vi "Close Notifiers.vi"(8 "error in":errorcluster, 11 "Notifiers":T1) -> (0 "error out":errorcluster)   [LabVIEW 2015, in "Notifiers.lvlib"]
doc: "Releases notifiers"
uses:
  Notifiers.lvlib
  Notifiers.ctl
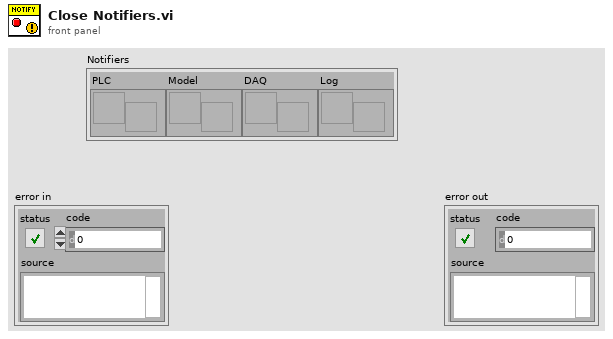
[diagram p1: front panel]
types:
  T1 = typedef "Notifiers.lvlib/Notifiers.ctl" = cluster{"PLC":refnum<notifier>, "Model":refnum<notifier>, "DAQ":refnum<notifier>, "Log":refnum<notifier>}
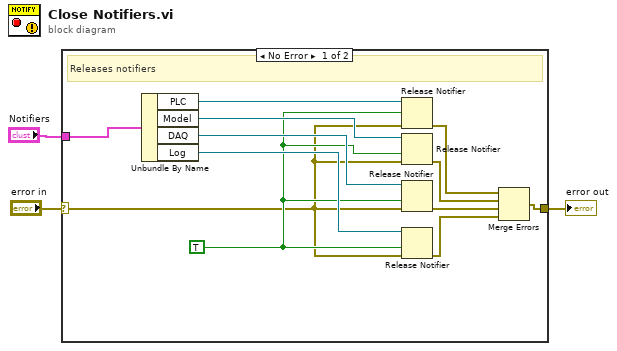
[diagram p0: block diagram]
diagram:
  n1 = case shown="No Error" "error in" {
    selector: "error in" -> [w4 w16]
    tunnel: [w12 w16] -> w2
    tunnel: "Notifiers" -> [w15 _]
    frame No Error {
      w5 = TRUE ("force destroy? (F)")
      # "Releases notifiers"
      n2 = Unbundle By Name(w15) -> ("PLC"=w14:refnum<notifier>, "Model"=w11:refnum<notifier>, "DAQ"=w9:refnum<notifier>, "Log"=w6:refnum<notifier>)
      n3 = Release Notifier(notifier=w14, force destroy? (F)=w5, error in (no error)=w4) -> (error out=w13:errorcluster)  [unwired: 2 out]
      n4 = Release Notifier(notifier=w11, force destroy? (F)=w5, error in (no error)=w4) -> (error out=w10:errorcluster)  [unwired: 2 out]
      n5 = Release Notifier(notifier=w9, force destroy? (F)=w5, error in (no error)=w4) -> (error out=w8:errorcluster)  [unwired: 2 out]
      n6 = Release Notifier(notifier=w6, force destroy? (F)=w5, error in (no error)=w4) -> (error out=w7:errorcluster)  [unwired: 2 out]
      n7 = Merge Errors(w13, w10, w8, w7) -> (w12:errorcluster)
    }
    frame Error {
    }
  }
  "error out" <- w2
